vi "to_turns.vi"(8 "Radio Buttons":enum32{"run valve", "bypass valve"}(radio), 11 "Steps":i32) -> (3 "Turns":dbl)   [LabVIEW 2015]
uses:
  global_motor.vi
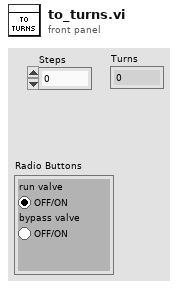
[diagram p1: front panel]
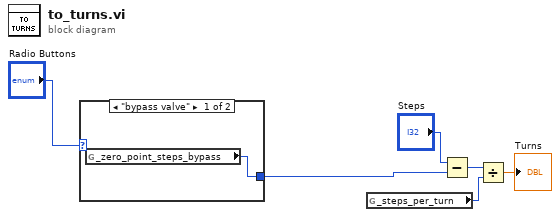
[diagram p0: block diagram]
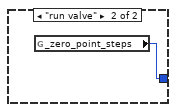
[diagram p2: hidden frame]
diagram:
  n1 = case shown="\"bypass valve\"" "Radio Buttons" {
    tunnel: [w7 w8] -> w2
    frame "bypass valve" {
      n2 = global read "global_motor.vi" "_zero_point_steps_bypass"() -> (w7:i32)
    }
    frame "run valve" {
      n3 = global read "global_motor.vi" "_zero_point_steps"() -> (w8:i32)
    }
  }
  n4 = global read "global_motor.vi" "_steps_per_turn"() -> (w3:i32)
  n5 = Subtract(x="Steps", y=w2) -> (x-y=w5:i32)
  n6 = Divide(x=w5, y=w3) -> (x/y=→"Turns":dbl)
